vi "write_attributes.vi"(8 "error in (no error)":errorcluster caption="entrée d'erreur (pas d'erreur)", 10 "attributes":T1, 11 "AffinityPropagation en entrée":refnum<class "AffinityPropagation.lvclass">) -> (0 "error out":errorcluster caption="sortie d'erreur", 3 "AffinityPropagation en sortie":refnum<class "AffinityPropagation.lvclass">)   [LabVIEW 2020, in "AffinityPropagation.lvclass"]
uses:
  AffinityPropagation.lvclass
  Controls/affinity_propagation_attributes.ctl
  AffinityPropagation.lvclass/AffinityPropagation.ctl
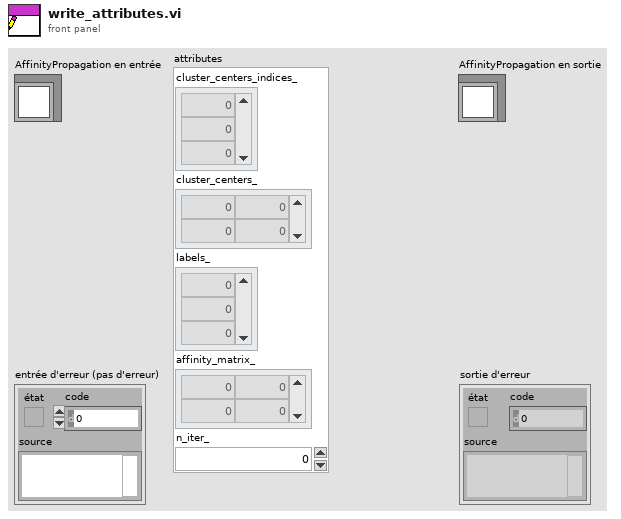
[diagram p1: front panel]
types:
  T1 = typedef "affinity_propagation_attributes.ctl" = cluster{"cluster_centers_indices_":dbl[], "cluster_centers_":dbl[][], "labels_":dbl[], "affinity_matrix_":dbl[][], "n_iter_":dbl}
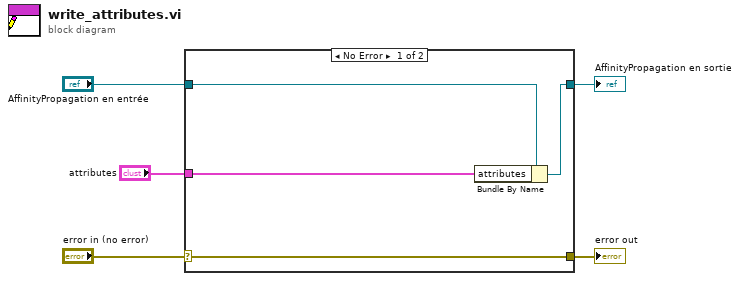
[diagram p0: block diagram]
diagram:
  n1 = case shown="No Error" "error in (no error)" {
    selector: "error in (no error)" -> [w9 w10]
    tunnel: [w9 w10] -> w4
    tunnel: [w7 w11] -> w2
    tunnel: "AffinityPropagation en entrée" -> [w8 w11]
    tunnel: "attributes" -> [w6 _]
    frame No Error {
      n2 = Bundle By Name(cluster=w8, "attributes"=w6) -> (w7:refnum<class "AffinityPropagation.lvclass">)
    }
    frame Error {
    }
  }
  "error out" <- w4
  "AffinityPropagation en sortie" <- w2
